vi "Data Save Timer.vi"(0 "delay(ms)":u32, 2 "Init(1)":i32=1) -> (4 "time up?":bool, 8 "first time?":bool, 15 "Time Left":u32)   [LabVIEW 2018]
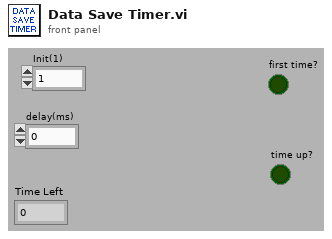
[diagram p1: front panel]
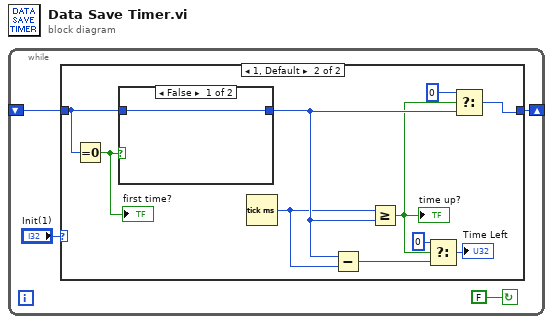
[diagram p0: block diagram]
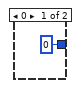
[diagram p2: hidden frame]
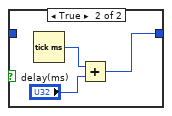
[diagram p3: hidden frame]
diagram:
  n1 = while {
    shift-right: [w3] -> _
    shift-left: _ -> [w2]
    stop <- FALSE continue-if-true
    n2 = case shown="1, Default" "Init(1)" {
      tunnel: [u32 0 ("millisecond timer value") w12] -> w3
      tunnel: w2 -> [_ w14]
      frame 0 {
      }
      frame 1, Default {
        n3 = Equal To 0?(x=w14) -> (x = 0?=w15:bool)
        "first time?" <- w15
        n4 = case shown="False" w15 {
          tunnel: [w16 w17] -> w11
          tunnel: w14 -> [w16 _]
          frame False {
          }
          frame True {
            n5 = Tick Count (ms)() -> (millisecond timer value=w18:u32)
            n6 = Add(x=w18, y="delay(ms)") -> (x+y=w17:u32)
          }
        }
        n7 = Tick Count (ms)() -> (millisecond timer value=w10:u32)
        n8 = Subtract(x=w11, y=w10) -> (x-y=w7:u32)
        n9 = Greater Or Equal?(x=w10, y=w11) -> (x >= y?=w8:bool)
        "time up?" <- w8
        n10 = Select(t=u32 0, s=w8, f=w7) -> (s? t:f=→"Time Left":u32)
        n11 = Select(t=u32 0, s=w8, f=w11) -> (s? t:f=w12:u32)
      }
    }
  }
